vi "Wait on Target.vi"(8 "error in (no error)":errorcluster, 10 "timeout in ms (-1)":i32, 11 "Queue in":refnum<queue>) -> (0 "error out":errorcluster, 1 "timed out?":bool, 2 "targets":T1[](array[typedef]), 3 "capturedAgoMs":i32)   [LabVIEW 2016, in "Vision Server.lvclass"]
uses:
  Vision Server.lvclass
  typedef/Target Vector.ctl
  typedef/Target Message JSON.ctl
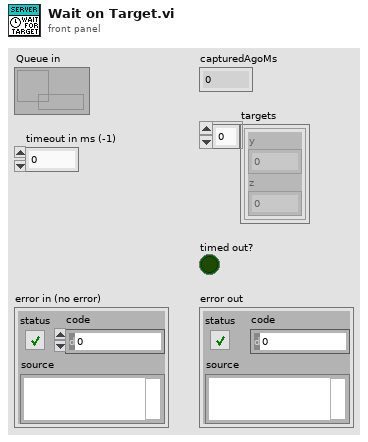
[diagram p1: front panel]
types:
  T1 = typedef "Vision Server.lvclass/Target Vector.ctl" = cluster{"y":dbl, "z":dbl}
  T2 = typedef "Vision Server.lvclass/Target Message JSON.ctl" = cluster{"capturedAgoMs":i32, "targets":T1[]}
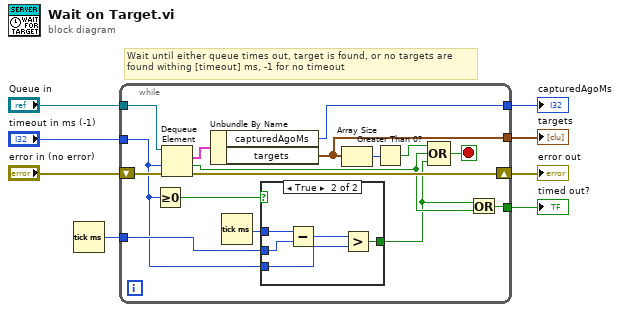
[diagram p0: block diagram]
diagram:
  # "Wait until either queue times out, target is found, or no targets are found withing [timeout] ms, -1 for no timeout"
  n1 = Tick Count (ms)() -> (millisecond timer value=w1:u32)
  n2 = while {
    tunnel: [w10] -> w7
    tunnel: "timeout in ms (-1)" -> [w12]
    tunnel: [w19] -> w6
    tunnel: [w23] -> w5
    tunnel: "Queue in" -> [w21]
    shift-right: [w24] -> w8
    shift-left: "error in (no error)" -> [w20]
    tunnel: w1 -> [w14]
    stop <- w17 stop-if-true
    n3 = Greater Or Equal To 0?(x=w12) -> (x >= 0?=w13:bool)
    n4 = Dequeue Element(queue=w21, timeout in ms (-1)=w12, error in (no error)=w20) -> (element=w22:T2, timed out?=w15:bool, error out=w24:errorcluster)  [unwired: 1 out]
    n5 = Unbundle By Name(w22) -> ("capturedAgoMs"=w23:i32, "targets"=w19:T1[])
    n6 = Tick Count (ms)() -> (millisecond timer value=w11:u32)
    n7 = case shown="True" w13 {
      tunnel: w11 -> [_ w29]
      tunnel: w14 -> [_ w28]
      tunnel: [_ w26] -> w9
      tunnel: w12 -> [_ w25]
      frame False {
      }
      frame True {
        n8 = Subtract(x=w29, y=w28) -> (x-y=w27:u32)
        n9 = Greater?(x=w27, y=w25) -> (0:w26:bool)
      }
    }
    n10 = Array Size(array=w19) -> (size(s)=w18:i32)
    n11 = Greater Than 0?(x=w18) -> (x > 0?=w16:bool)
    n12 = Compound Arithmetic op=OR(w16, w15, w9) -> (w17:bool)
    n13 = Or(x=w9, y=w15) -> (x .or. y?=w10:bool)
  }
  "timed out?" <- w7
  "error out" <- w8
  "targets" <- w6
  "capturedAgoMs" <- w5
